vi "ZLockConnect.vi"(7 "context (create new)":T1 format="%.0x", 8 "error in (no error)":errorcluster, 9 "port (7339)":i32=7339, 10 "host":string="130.194.5.78", 11 "ZLock in":refnum<class "ZLock.lvclass">) -> (0 "error out":errorcluster, 3 "ZLock out":refnum<class "ZLock.lvclass">)   [LabVIEW 2012, in "ZLock.lvclass"]
uses:
  <userlib>/BIAS2/subvis/zlock/ZLock.lvclass
  <vilib>/addons/zeromq/pointer.ctl
  <userlib>/BIAS2/subvis/zlock/ZLock.lvclass/ZLock.ctl
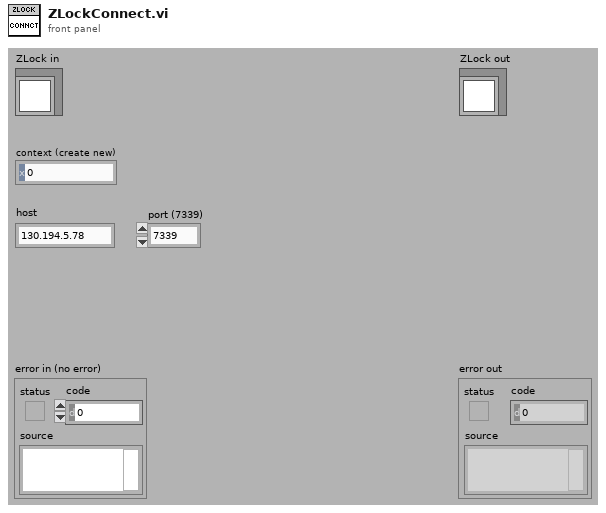
[diagram p1: front panel]
types:
  T1 = typedef "pointer.ctl" = u64
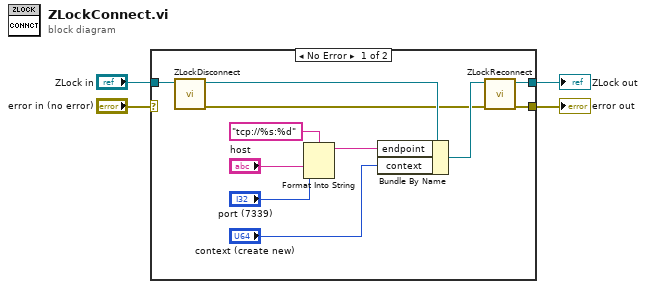
[diagram p0: block diagram]
diagram:
  n1 = case shown="No Error" "error in (no error)" {
    selector: "error in (no error)" -> [_ w17]
    tunnel: [w6 w17] -> w3
    tunnel: [w8 w16] -> w1
    tunnel: "ZLock in" -> [w11 w16]
    frame No Error {
      n2 = call-dynamic "ZLockDisconnect.vi"("ZLock in"=w11) -> ("error out"=w5:errorcluster, "ZLock out"=w9:refnum<class "ZLock.lvclass">)  [unwired: 9 in]
      n3 = Format Into String(format string="tcp://%s:%d", "host", "port (7339)") -> (resulting string=w12:string)  [unwired: 2 in, 1 out]
      n4 = Bundle By Name(cluster=w9, "endpoint"=w12, "context"="context (create new)") -> (w10:refnum<class "ZLock.lvclass">)
      n5 = call-dynamic "ZLockReconnect.vi"("error in (no error)"=w5, "ZLock in"=w10) -> ("error out"=w6:errorcluster, "ZLock out"=w8:refnum<class "ZLock.lvclass">)  [unwired: 8 in]
    }
    frame Error {
    }
  }
  "error out" <- w3
  "ZLock out" <- w1
